vi "create_timing_chart.vi"() -> ()   [LabVIEW 2011]
uses:
  <vilib>/Waveform/DWDTOps.llb/DWDT Boolean Array to Digital.vi
panel:
  in  "G duration":dbl=1.0 min=0.0 format="%_5g"
  in  "G":dbl min=0.0 format="%_5g"
  in  "E duration":dbl=1.0 min=0.0 format="%_5g"
  in  "E":dbl min=0.0 format="%_5g"
  in  "C duration":dbl=1.0 min=0.0 format="%_5g"
  in  "C":dbl min=0.0 format="%_5g"
  in  "A duration":dbl=1.0 min=0.0 format="%_5g"
  in  "A":dbl min=0.0 format="%_5g"
  in  "overall length [ms]":dbl=1000.0
  in  "t0 duration":dbl=1.0 min=0.0 format="%_5g"
  in  "t0":dbl min=0.0 format="%_5g"
  out "Digital Waveform Graph":digitalwaveform(graph)
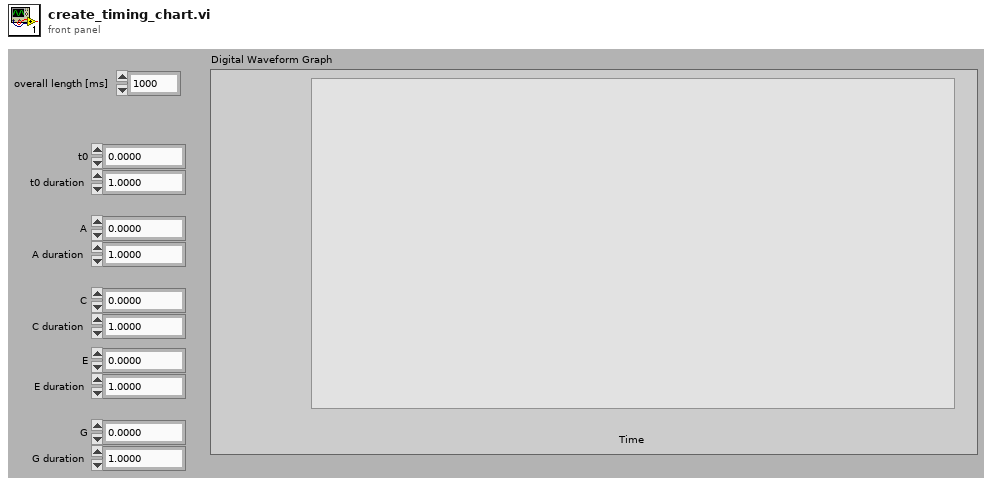
[diagram p1: front panel]
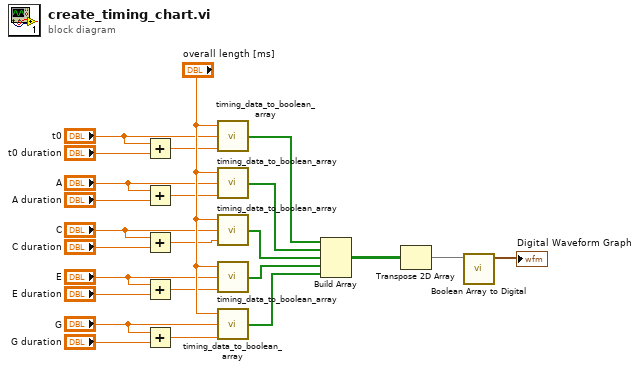
[diagram p0: block diagram]
diagram:
  n1 = Add(x="t0", y="t0 duration") -> (x+y=w5:dbl)
  n2 = Add(x="A", y="A duration") -> (x+y=w4:dbl)
  n3 = Add(x="C", y="C duration") -> (x+y=w3:dbl)
  n4 = Add(x="E", y="E duration") -> (x+y=w2:dbl)
  n5 = Add(x="G", y="G duration") -> (x+y=w1:dbl)
  n6 = call "timing_data_to_boolean_array.vi"("end time [us]"=w5, "start time [us]"="t0", "overall length [us]"="overall length [ms]") -> ("boolean timing array"=w21:bool[])  [unwired: 1 in]
  n7 = call "timing_data_to_boolean_array.vi"("end time [us]"=w4, "start time [us]"="A", "overall length [us]"="overall length [ms]") -> ("boolean timing array"=w11:bool[])  [unwired: 1 in]
  n8 = call "timing_data_to_boolean_array.vi"("end time [us]"=w3, "start time [us]"="C", "overall length [us]"="overall length [ms]") -> ("boolean timing array"=w14:bool[])  [unwired: 1 in]
  n9 = call "timing_data_to_boolean_array.vi"("end time [us]"=w2, "start time [us]"="E", "overall length [us]"="overall length [ms]") -> ("boolean timing array"=w13:bool[])  [unwired: 1 in]
  n10 = call "timing_data_to_boolean_array.vi"("end time [us]"=w1, "start time [us]"="G", "overall length [us]"="overall length [ms]") -> ("boolean timing array"=w12:bool[])  [unwired: 1 in]
  n11 = Build Array(w21, w11, w14, w13, w12) -> (w23:bool[][])
  n12 = Transpose 2D Array(2D array=w23) -> (transposed array=w22:bool[][])
  n13 = call-poly <vilib>:"Boolean Array to Digital.vi"("boolean array"=w22) -> ("digital waveform"=→"Digital Waveform Graph":digitalwaveform)  [unwired: 9 in, 1 out]
